vi "toOCU.vi"(8 "error in (no error)":errorcluster, 9 "Mission Notifiers":T1, 10 "NotifierReff":T2, 11 "NetworkStreamWriter in":refnum<class "NetworkStreamWriter.lvclass">) -> (0 "error out":errorcluster, 3 "NetworkStreamWriter out":refnum<class "NetworkStreamWriter.lvclass">)   [LabVIEW 2013]
doc: "writes all notifiers to OCU when they're updated\n\nImportaint: when new notifiers are created, this VI must be updated. For doubles, booleans, and double arrays, simply add them to the appropriate unbundle category. For anything else, add them to the \"other\" category and copy the code from the others.\n\nKaitlin Gallagher\n3/4/14"
uses:
  RIO-OCU_Comm/NetworkStreams/Writer/NetworkStreamWriter.lvclass
  Data/TypeDefs/Notifiers.ctl
  Data/TypeDefs/UTM Location.ctl
  Data/TypeDefs/Sail Set Suggestions.ctl
  Data/TypeDefs/Rudder Set Suggestions.ctl
  Data/TypeDefs/OverrideInformation.ctl
  Data/TypeDefs/OverrideMode.ctl
  Data/TypeDefs/MotorSetup.ctl
  Data/TypeDefs/DynamixelSetupInfo.ctl
  Data/TypeDefs/AirmarStatus.ctl
  Data/TypeDefs/HardwareOnline.ctl
  Data/TypeDefs/DynamixelCycleTracker.ctl
  Data/TypeDefs/RC Input Values.ctl
  Classes/Waypoint/Waypoint.lvclass
  Data/TypeDefs/MissionNotifiers.ctl
  Classes/Missions/GenericMission/GenericMission.lvclass
  Classes/Obstacle/Obstacle.lvclass
panel:
  # "Disabled"
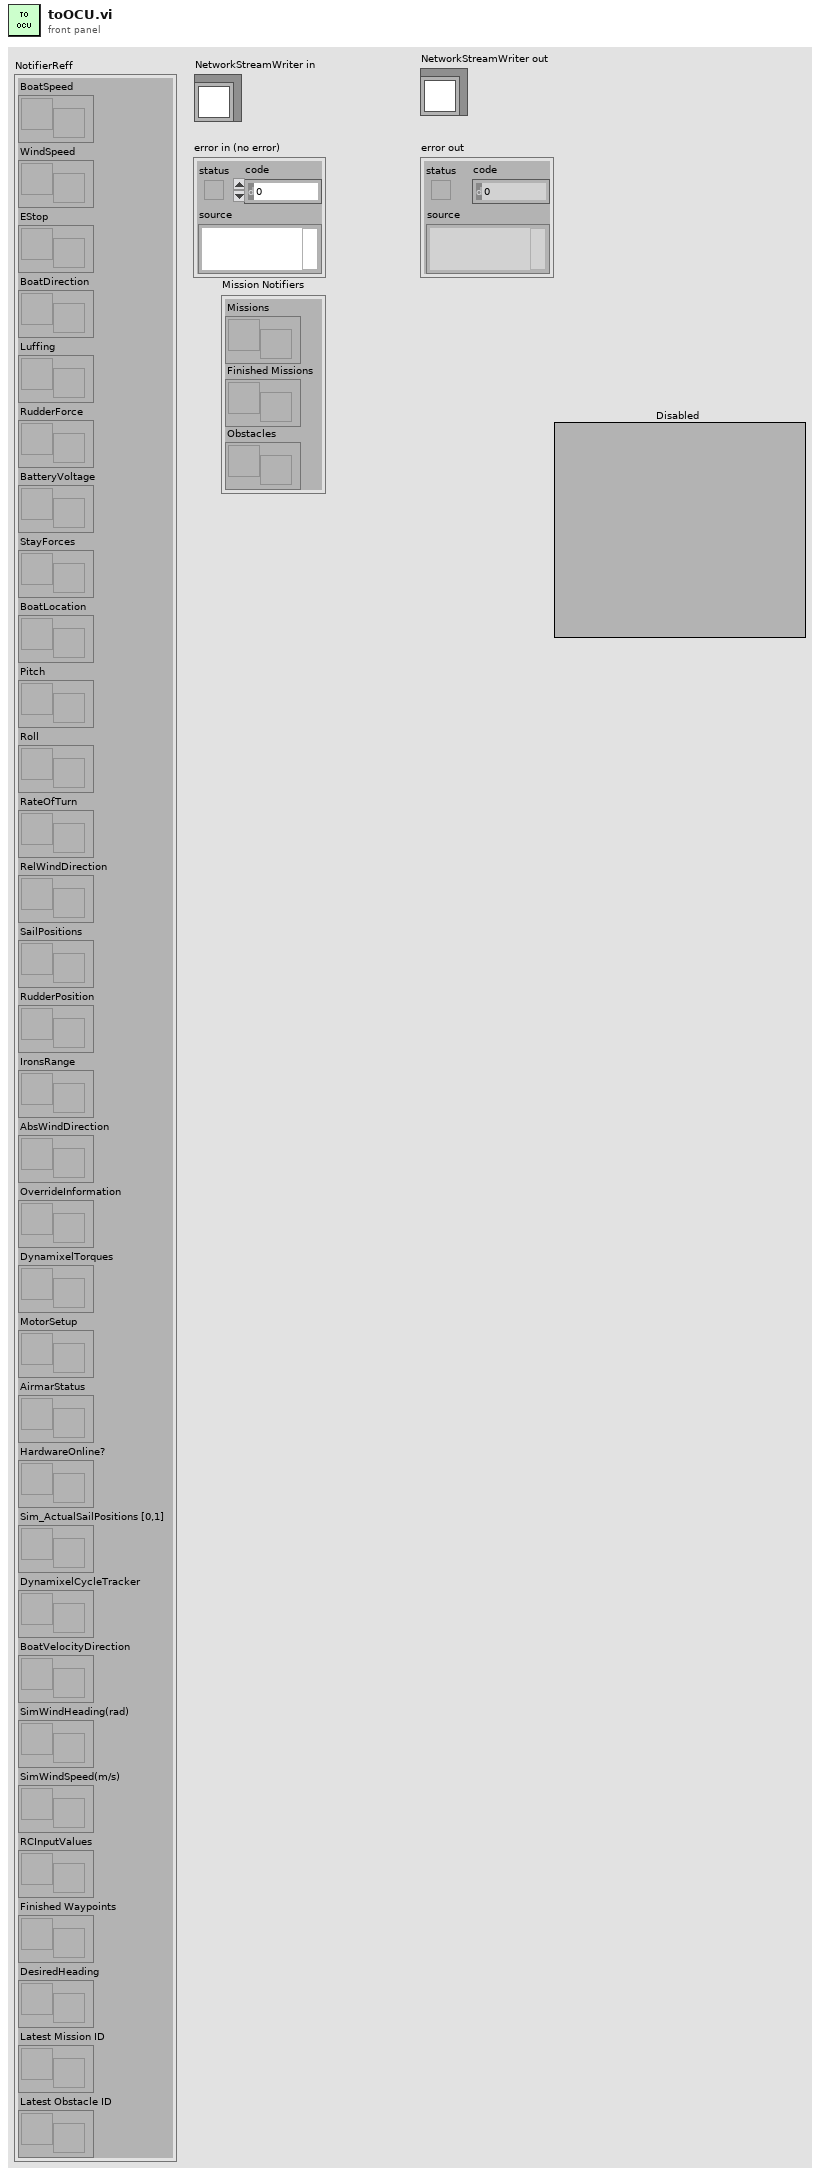
[diagram p1: front panel]
types:
  T1 = typedef "MissionNotifiers.ctl" = cluster{"Missions":refnum<notifier>, "Finished Missions":refnum<notifier>, "Obstacles":refnum<notifier>}
  T2 = typedef "Notifiers.ctl" = cluster{"BoatSpeed":refnum<notifier>, "WindSpeed":refnum<notifier>, "EStop":refnum<notifier>, "BoatDirection":refnum<notifier>, "Luffing":refnum<notifier>, "RudderForce":refnum<notifier>, "BatteryVoltage":refnum<notifier>, "StayForces":refnum<notifier>, "BoatLocation":refnum<notifier>, "Pitch":refnum<notifier>, "Roll":refnum<notifier>, "RateOfTurn":refnum<notifier>, "RelWindDirection":refnum<notifier>, "SailPositions":refnum<notifier>, "RudderPosition":refnum<notifier>, "IronsRange":refnum<notifier>, "AbsWindDirection":refnum<notifier>, "OverrideInformation":refnum<notifier>, "DynamixelTorques":refnum<notifier>, "MotorSetup":refnum<notifier>, "AirmarStatus":refnum<notifier>, "HardwareOnline?":refnum<notifier>, "Sim_ActualSailPositions [0,1]":refnum<notifier>, "DynamixelCycleTracker":refnum<notifier>, "BoatVelocityDirection":refnum<notifier>, "SimWindHeading(rad)":refnum<notifier>, "SimWindSpeed(m/s)":refnum<notifier>, "RCInputValues":refnum<notifier>, "Finished Waypoints":refnum<notifier>, "DesiredHeading":refnum<notifier>, "Latest Mission ID":refnum<notifier>, "Latest Obstacle ID":refnum<notifier>}
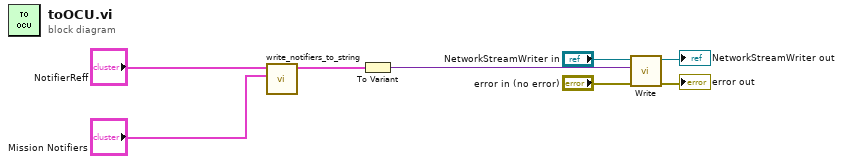
[diagram p0: block diagram]
diagram:
  n1 = call "write_notifiers_to_string.vi"("Mission Notifiers"="Mission Notifiers", "NotifierReff"="NotifierReff") -> ("input cluster"=w3:cluster{"names":string, "value":variant})  [unwired: 9 in]
  n2 = To Variant(anything=w3) -> (Variant=w4:variant)
  n3 = call "Write.vi"("error in (no error)"="error in (no error)", "element"=w4, "NetworkStreamWriter in"="NetworkStreamWriter in") -> ("error out"=→"error out":errorcluster, "NetworkStreamWriter out"=→"NetworkStreamWriter out":refnum<class "NetworkStreamWriter.lvclass">)  [unwired: 7 in]
